vi "Build md5.vi"(8 "error in (no error)":errorcluster, 9 "suffix":string, 10 "words":string, 11 "prefix":string) -> (0 "error out":errorcluster, 3 "MD5 Message Digest":string)   [LabVIEW 2016]
uses:
  <userlib>/_OpenG.lib/md5/md5.llb/MD5 Message Digest (Binary String)__ogtk.vi
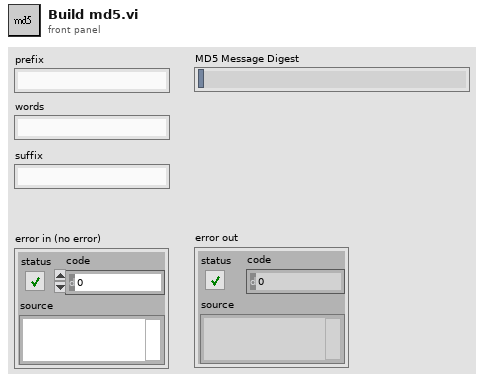
[diagram p1: front panel]
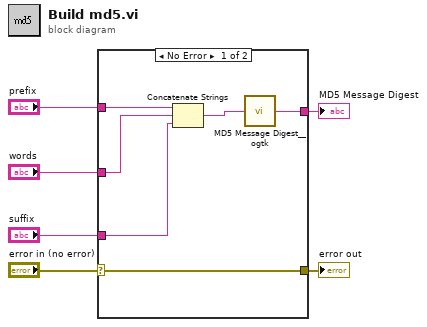
[diagram p0: block diagram]
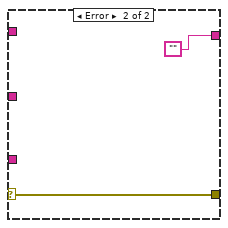
[diagram p2: hidden frame]
diagram:
  n1 = case shown="No Error" "error in (no error)" {
    selector: "error in (no error)" -> [w9 w14]
    tunnel: "suffix" -> [w7 _]
    tunnel: "prefix" -> [w11 _]
    tunnel: [w10 ""] -> w4
    tunnel: [w9 w14] -> w2
    tunnel: "words" -> [w8 _]
    frame No Error {
      n2 = Concatenate Strings(w11, w8, w7) -> (w12:string)
      n3 = call-poly <userlib>:"MD5 Message Digest__ogtk.vi"("Message"=w12) -> ("MD5 Message Digest"=w10:string)
    }
    frame Error {
    }
  }
  "MD5 Message Digest" <- w4
  "error out" <- w2
